vi "ComputeVector.vi"(0 "Image":T1, 4 "error in":errorcluster, 6 "Matches":T2(array[cluster]), 7 "Color":u32(colorbox)=16711680) -> (13 "error out":errorcluster, 14 "Image Out":T1, 16 "X Pixel":dbl, 17 "Y Pixel":dbl, 18 "X (um)":dbl format="%#_4g", 19 "Y (um)":dbl format="%#_4g")   [LabVIEW 2019]
uses:
  <vilib>/vision/Image Controls.llb/IMAQ Image.ctl
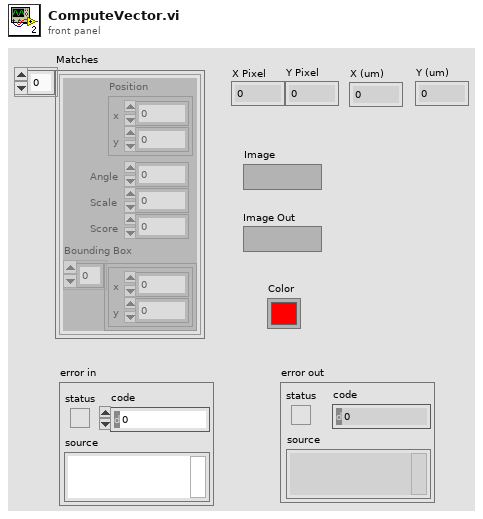
[diagram p1: front panel]
types:
  T1 = typedef "IMAQ Image.ctl" = refnum<image>
  T2 = cluster{"Position":cluster{"x":sgl, "y":sgl}, "Angle":sgl, "Scale":sgl, "Score":sgl, "Bounding Box":cluster{"x":sgl, "y":sgl}[]}[]
  T3 = cluster{"Position":cluster{"x":sgl, "y":sgl}, "Angle":sgl, "Scale":sgl, "Score":sgl, "Bounding Box":cluster{"x":sgl, "y":sgl}[]}
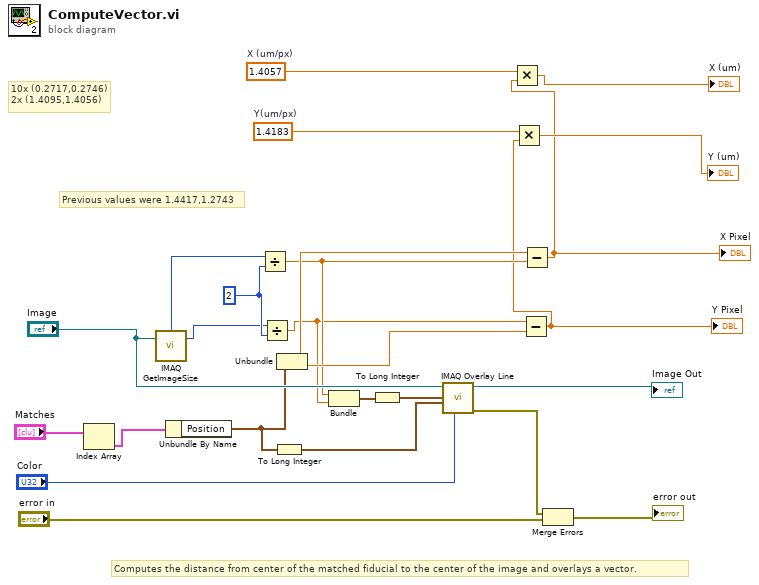
[diagram p0: block diagram]
diagram:
  w1 = 1.4183  # Y(um/px)
  w2 = 1.4057  # X (um/px)
  w22 = 2
  # "10x (0.2717,0.2746)\n2x (1.4095,1.4056)"
  # "Previous values were 1.4417,1.2743"
  # "Computes the distance from center of the matched fiducial to the center of the image and overlays a vector."
  n1 = Index Array(array="Matches") -> (element=w14:T3)  [unwired: 1 in]
  n2 = call "IMAQ GetImageSize"("Image"="Image") -> ("Y Resolution"=w7:i32, "X Resolution"=w8:i32)  [unwired: 3 in, 1 out]
  n3 = Unbundle By Name(w14) -> ("Position"=w19:cluster{"x":sgl, "y":sgl})
  n4 = Divide(x=w8, y=w22) -> (x/y=w11:dbl)
  n5 = Divide(x=w7, y=w22) -> (x/y=w10:dbl)
  n6 = To Long Integer(number=w19) -> (32bit integer=w18:cluster{"x":i32, "y":i32})
  n7 = Unbundle(w19) -> ("x"=w20:sgl, "y"=w21:sgl)
  n8 = Bundle(w11, w10) -> (w9:cluster{dbl, dbl})  [unwired: 1 in]
  n9 = To Long Integer(number=w9) -> (32bit integer=w17:cluster{i32, i32})
  n10 = call "IMAQ Overlay Line"("Color"="Color", "End Point"=w18, "Start Point"=w17, "Image"="Image") -> ("error out"=w16:errorcluster, "Image Out"=→"Image Out":T1)  [unwired: 6 in]
  n11 = Subtract(x=w10, y=w21) -> (x-y=w4:dbl)
  "Y Pixel" <- w4
  n12 = Multiply(x=w1, y=w4) -> (x*y=→"Y (um)":dbl)
  n13 = Subtract(x=w20, y=w11) -> (x-y=w3:dbl)
  "X Pixel" <- w3
  n14 = Multiply(x=w2, y=w3) -> (x*y=→"X (um)":dbl)
  n15 = Merge Errors(w16, "error in") -> (→"error out":errorcluster)
